vi "LogFudgerData.vi"(6 "Run Ratios":T2 {"LEC13/12" format="%_4e"; "DTfrac" format="%#_3g"; "DT" format="%#_3g"; "CountErr" format="%#_3g"; "d13C" format="%_4g"; "C13/12" format="%_4e"; "C14/12" format="%_4e"; "C14/13" format="%_3e"; "C12Cor" format="%_3e"; "C13" format="%_3e"; "C13H/L" format="%#_3g"}, 8 "error in (no error)":errorcluster, 9 "Run Summary":T3 {"C12LE" format="%_3e"; "C13LE" format="%_3e"; "C1312" format="%_3e"; "C12" format="%_3e"; "C13L" format="%_3e"; "C13H" format="%_3e"}, 10 "Sample Data":T1, 11 "Log File Path":path) -> (0 "error out":errorcluster, 1 "Result string":string)   [LabVIEW 2013]
uses:
  ctl/SummaryData.ctl
  ctl/RunRatios.ctl
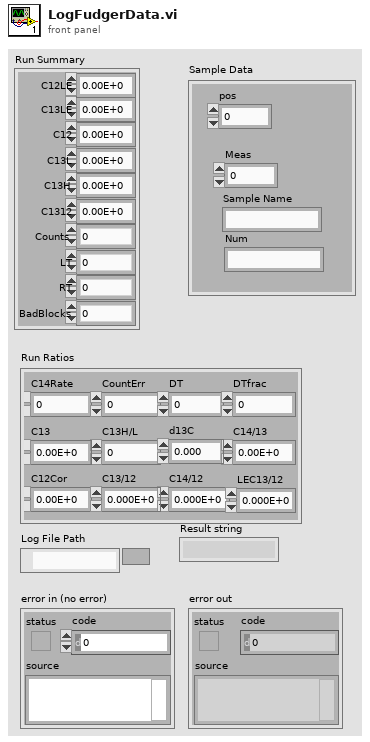
[diagram p1: front panel]
types:
  T1 = cluster{"pos":i32, "Meas":i32, "Sample Name":string, "Num":string}
  T2 = typedef "RunRatios.ctl" = cluster{"C14Rate":dbl, "CountErr":dbl, "DT":dbl, "DTfrac":dbl, "C13":dbl, "C13H/L":dbl, "d13C":dbl, "C14/13":dbl, "C12Cor":dbl, "C13/12":dbl, "C14/12":dbl, "LEC13/12":dbl}
  T3 = typedef "SummaryData.ctl" = cluster{"C12LE":dbl, "C13LE":dbl, "C12":dbl, "C13L":dbl, "C13H":dbl, "C1312":dbl, "Counts":u32, "LT":dbl, "RT":dbl, "BadBlocks":u8}
  T4 = enum16{"open", "replace", "create", "open or create", "replace or create", "replace or create with confirmation"}
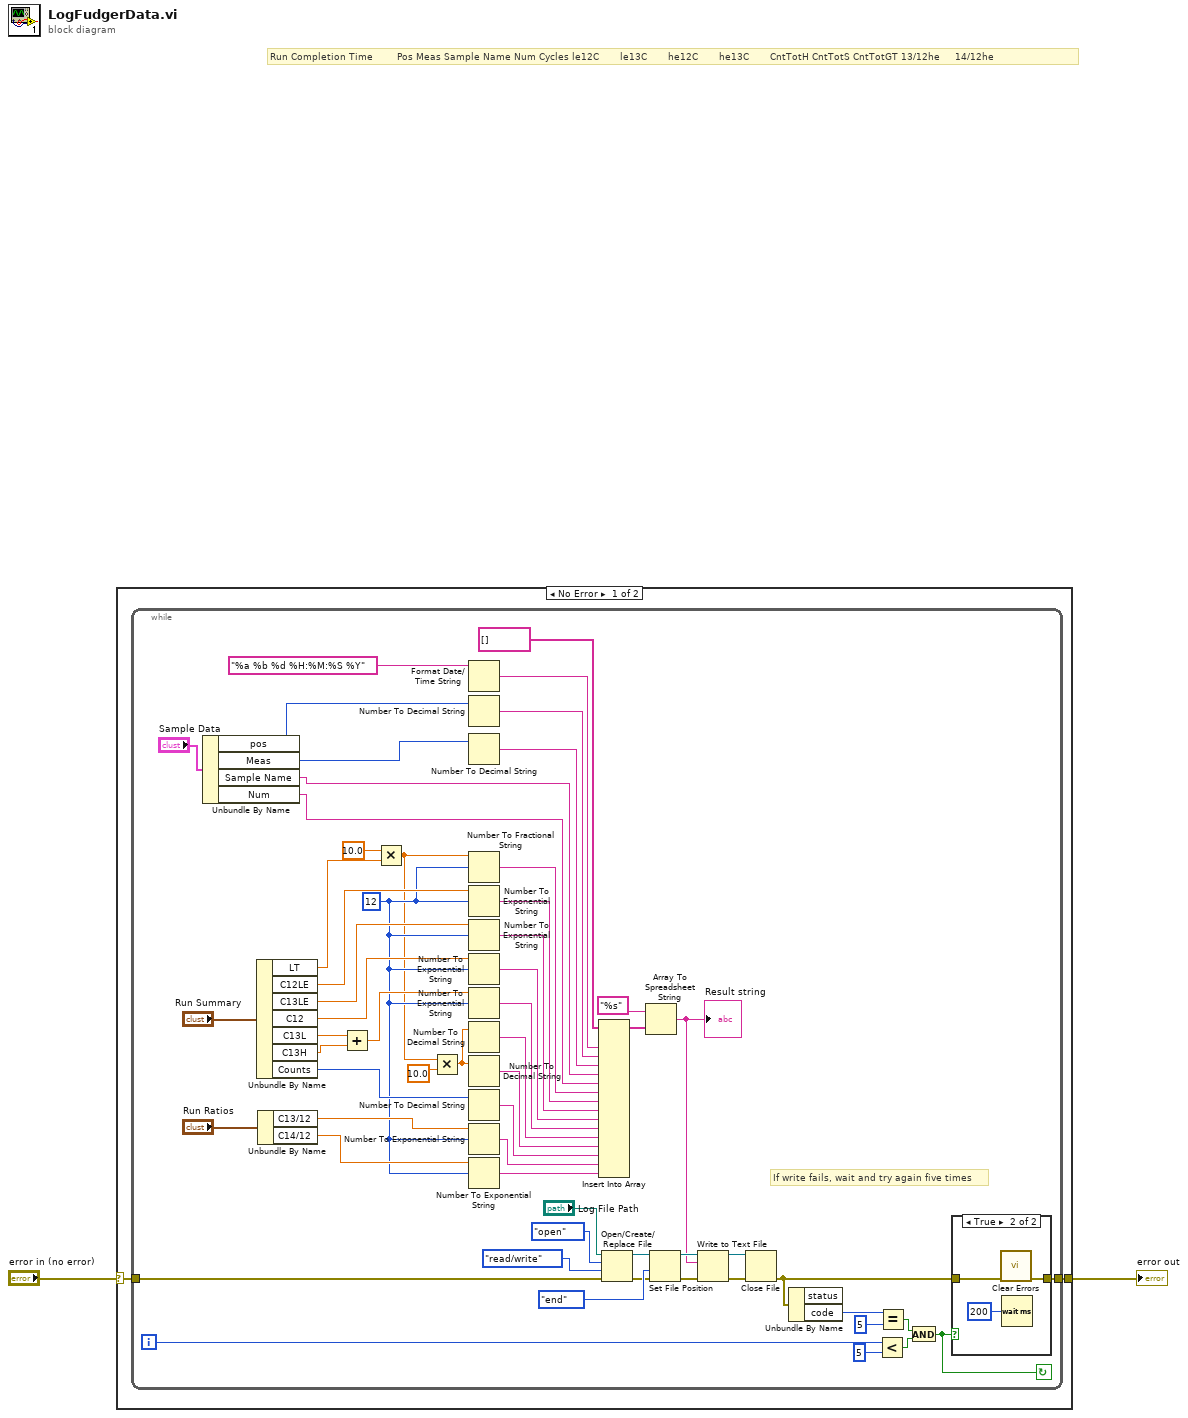
[diagram p0: block diagram]
diagram:
  # "Run Completion Time       \tPos\tMeas\tSample Name\tNum\tCycles\tle12C      \tle13C      \the12C      \the13C      \tCntTotH\tCntTotS\tCntTotGT\t13/12he    \t14/12he"
  n1 = case shown="No Error" "error in (no error)" {
    selector: "error in (no error)" -> [w4 w69]
    tunnel: [w3 w69] -> w1
    frame No Error {
      n2 = while {
        tunnel: w4 -> [w25]
        tunnel: [w7] -> w3
        i -> [w12]
        stop <- w9 continue-if-true
        w19 = i16 12 ("width (-)")
        # "If write fails, wait and try again five times"
        n3 = Unbundle By Name("Sample Data") -> ("pos"=w21:i32, "Meas"=w5:i32, "Sample Name"=w20:string, "Num"=w6:string)
        n4 = Unbundle By Name("Run Summary") -> ("LT"=w23:dbl, "C12LE"=w38:dbl, "C13LE"=w37:dbl, "C12"=w36:dbl, "C13L"=w35:dbl, "C13H"=w34:dbl, "Counts"=w32:u32)
        n5 = Unbundle By Name("Run Ratios") -> ("C13/12"=w30:dbl, "C14/12"=w29:dbl)
        n6 = Add(x=w35, y=w34) -> (x+y=w33:dbl)
        n7 = Multiply(x=10.0, y=w23) -> (x*y=w17:dbl)
        n8 = Multiply(x=w17, y=10.0) -> (x*y=w16:dbl)
        n9 = Format Date/Time String(time format string (%c)="%a %b %d %H:%M:%S %Y") -> (date/time string=w63:string)  [unwired: 2 out]
        n10 = Number To Decimal String(number=w21) -> (decimal integer string=w53:string)  [unwired: 1 out]
        n11 = Number To Decimal String(number=w5) -> (decimal integer string=w52:string)  [unwired: 1 out]
        n12 = Number To Fractional String(number=w17, width (-)=w19) -> (F-format string=w51:string)  [unwired: 2 in]
        n13 = Number To Exponential String(number=w38, 3:w19) -> (E-format string=w50:string)  [unwired: 2 in]
        n14 = Number To Exponential String(number=w37, 3:w19) -> (E-format string=w49:string)  [unwired: 2 in]
        n15 = Number To Exponential String(number=w36, 3:w19) -> (E-format string=w48:string)  [unwired: 2 in]
        n16 = Number To Exponential String(number=w33, 3:w19) -> (E-format string=w47:string)  [unwired: 2 in]
        n17 = Number To Decimal String(number=w16) -> (decimal integer string=w46:string)  [unwired: 1 out]
        n18 = Number To Decimal String(number=w16) -> (decimal integer string=w45:string)  [unwired: 1 out]
        n19 = Number To Decimal String(number=w32) -> (decimal integer string=w44:string)  [unwired: 1 out]
        n20 = Number To Exponential String(number=w30, 3:w19) -> (E-format string=w43:string)  [unwired: 2 in]
        n21 = Number To Exponential String(number=w29, 3:w19) -> (E-format string=w42:string)  [unwired: 2 in]
        n22 = Insert Into Array(array=string[] [], new element #1=w63, new element #2=w53, new element #3=w52, new element #4=w20, new element #5=w6, new element #6=w51, new element #7=w50, new element #8=w49, new element #9=w48, new element #10=w47, new element #11=w46, new element #12=w45, new element #13=w44, new element #14=w43, new element #15=w42) -> (w41:string[])  [unwired: 1 in]
        n23 = Open/Create/Replace File(file path (use dialog)="Log File Path", error in=w25, operation (0:open)=T4."open", access (0:read/write)=enum16{"read/write", "read-only", "write-only"}."read/write") -> (refnum out=w56:refnum<file>, error out=w28:errorcluster)  [unwired: 3 out]
        n24 = Array To Spreadsheet String(array=w41, 3:"%s" ("format string")) -> (spreadsheet string=w54:string)  [unwired: 1 out]
        "Result string" <- w54
        n25 = Set File Position(refnum=w56, from (0:start)=enum16{"start", "end", "current"}."end", error in=w28) -> (refnum out=w55:refnum<file>, error out=w27:errorcluster)  [unwired: 1 in]
        n26 = Write to Text File(file (use dialog)=w55, text=w54, error in=w27) -> (refnum out=w61:refnum<file>, error out=w26:errorcluster)  [unwired: 2 out]
        n27 = Close File(refnum=w61, error in=w26) -> (error out=w8:errorcluster)  [unwired: 1 out]
        n28 = Unbundle By Name(w8) -> ("code"=w15:i32)  [unwired: 1 out]
        n29 = Less?(x=w12, y=5) -> (x < y?=w13:bool)
        n30 = Equal?(x=w15, y=5) -> (x = y?=w10:bool)
        n31 = And(x=w10, y=w13) -> (x .and. y?=w9:bool)
        n32 = case shown="True" w9 {
          tunnel: [w65 w67] -> w7
          tunnel: w8 -> [w65 w66]
          frame False {
          }
          frame True {
            n33 = call <vilib>:"Clear Errors.vi"("error in (no error)"=w66) -> ("error out"=w67:errorcluster)  [unwired: 6 in]
            n34 = Wait (ms)(milliseconds to wait=u32 200) -> ()  [unwired: 1 out]
          }
        }
      }
    }
    frame Error {
    }
  }
  "error out" <- w1
